vi "Drive Controller.vi"(8 "error in":errorcluster) -> ()   [LabVIEW 2020]
doc: "This VI executes continuously carrying out the current operation and responding to updates or new operation requests. It will often contain the timing or control code that is difficult to place directly in TeleOp. This VI generally opens all sensors and motors and isolates the rest of the robot code from knowing implementation details of how the operations are carried out."
uses:
  Drive Setpoints.ctl
  Drive Operations.ctl
  Robot Velocities.ctl
  <vilib>/Rock Robotics/WPI/ThirdParty/Phoenix-LabVIEW/Motor Controller/Controls/CTRE_Phoenix_MotorControl_ControlMode.ctl
panel:
  in  "milliseconds to wait":u32
  out "Current\nCmd":string
  # "Tip: The graph shows the motor setpoints. It may also be helpful to observe inputs and sensor values.\nYou may also want to display tuning or debugging controls."
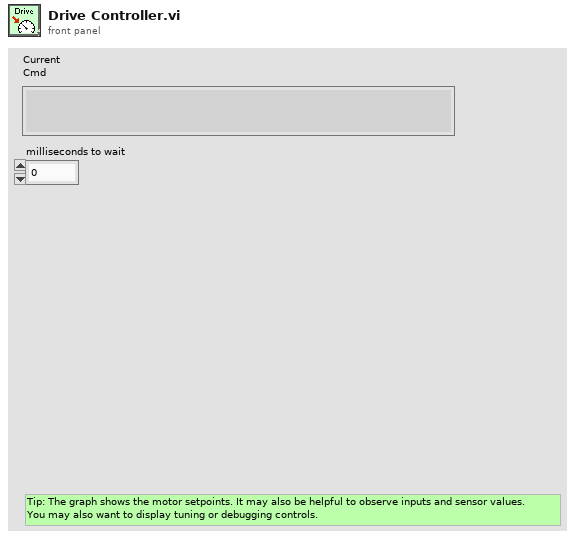
[diagram p1: front panel]
types:
  T1 = cluster{"LF radius":dbl[], "LB radius":dbl[], "RF radius":dbl[], "RB radius":dbl[]}
  T2 = cluster{"LF ID":u8, "LB ID":u8, "RF ID":u8, "RB ID":u8}
  T3 = typedef "Drive Setpoints.ctl" = cluster{"Operation":T4, "Robot Velocities":T5, "Reset Pods?":bool}
  T4 = typedef "Drive Operations.ctl" = enum16{"Reserve", "Read Current", "Immediate", "Calibrate"}
  T5 = typedef "Robot Velocities.ctl" = cluster{"vx":dbl, "vy":dbl, "w":dbl}
  T6 = typedef "Swerve Motors.ctl" = cluster{"Drive Motors":cluster{"Left Front":T7, "Left Back":T7, "Right Front":T7, "Right Back":T7}, "Steer Motors":cluster{"Left Front":T7, "Left Back":T7, "Right Front":T7, "Right Back":T7}}
  T7 = typedef "WPI_MotorControlDeviceRef.ctl" = cluster{"DeviceStatus":errorcluster, "Type":T8, "PWM":cluster{"PWM Channel":T9, "DeadBand":T10}, "CAN":cluster{"Device Number":u8, "SetOutput VI Ref":variant, "GetOutput VI Ref":variant, "Enable VI Ref":variant, "Disable VI Ref":variant, "Data":variant}, "Invert":bool, "DIO PWM":cluster{"PWM \"Enable\" Channel":T9, "DIOChannel":T11, "PWM Rate":dbl}}
  T8 = typedef "WPI_MotorControlType.ctl" = enum16{"PWM", "CAN", "DIO PWM"}
  T9 = typedef "FPGA_DIOPWMChannel.ctl" = enum8{"PWM 0", "PWM 1", "PWM 2", "PWM 3", "PWM 4", "PWM 5", "PWM 6", "PWM 7", "PWM 8", "PWM 9", "PWM MXP 0", "PWM MXP 1", "PWM MXP 2", "PWM MXP 3", "PWM MXP 4", "PWM MXP 5", "PWM MXP 6", "PWM MXP 7", "PWM MXP 8", "PWM MXP 9", "Invalid"}
  T10 = typedef "WPI_PWMDeadband.ctl" = cluster{"Name":string, "maxPositivePwm":i32, "minPositivePwm":i32, "centerPwm":i32, "maxNegativePwm":i32, "minNegativePwm":i32, "angularRange":u16}
  T11 = typedef "FPGA_DIOChannel.ctl" = enum8{"DIO 0", "DIO 1", "DIO 2", "DIO 3", "DIO 4", "DIO 5", "DIO 6", "DIO 7", "DIO 8", "DIO 9", "DIO MXP 0", "DIO MXP 1", "DIO MXP 2", "DIO MXP 3", "DIO MXP 4", "DIO MXP 5", "DIO MXP 6", "DIO MXP 7", "DIO MXP 8", "DIO MXP 9", "DIO MXP 10", "DIO MXP 11", "DIO MXP 12", "DIO MXP 13", "DIO MXP 14", "DIO MXP 15", "SPI Port CS1", "SPI Port CS2", "SPI Port CS3", "SPI Port MISO", "SPI Port MOSI", "Invalid"}
  T12 = typedef "Swerve CANCoders.ctl" = cluster{"Left Front":T13, "Left Back":T13, "Right Front":T13, "Right Back":T13}
  T13 = typedef "CTRE_Phoenix_CANcoder_DeviceRef.ctl" = cluster{"DeviceStatus":errorcluster, "Device Number":u8, "Handle":u64, "UsageFrame":u32, "Library Path":path}
  T14 = typedef "Command Status Info.ctl" = cluster{"Name":string, "Status":T15, "notifier out":T16}
  T15 = typedef "Completion Status.ctl" = enum16{"Successful", "Aborted", "Incomplete"}
  T16 = typedef "Completion Notifier.ctl" = refnum<notifier>
  T17 = cluster{"SubSystem Data":T3, cluster{"Start Time (ms)":u32, "Iterations":i32}, cluster{"Command Info":T14, "Description":string, "Default Command":T3, "queue out":refnum<queue>, "Subsystem Name":string}}
  T18 = cluster{"Left Front":dbl, "Left Back":dbl, "Right Front":dbl, "Right Back":dbl}
  T19 = cluster{"Left Front":i32, "Left Back":i32, "Right Front":i32, "Right Back":i32}
  T20 = typedef "Pod Setpoints.ctl" = cluster{"Left Front":cluster{"Velocity":dbl, "Theta":dbl}, "Left Back":cluster{"Velocity":dbl, "Theta":dbl}, "Right Front":cluster{"Velocity":dbl, "Theta":dbl}, "Right Back":cluster{"Velocity":dbl, "Theta":dbl}}
  T21 = typedef "CTRE_Phoenix_MotorControl_ControlMode.ctl" = u16
  T22 = cluster{"Left Front":T7, "Left Back":T7, "Right Front":T7, "Right Back":T7}
  T23 = cluster{"SubSystem Data":T3, cluster{"Start Time (ms)":u32, "Iterations":i32}, "Default Command Arguments":cluster{"Command Info":T14, "Description":string, "Default Command":T3, "queue out":refnum<queue>, "Subsystem Name":string}}
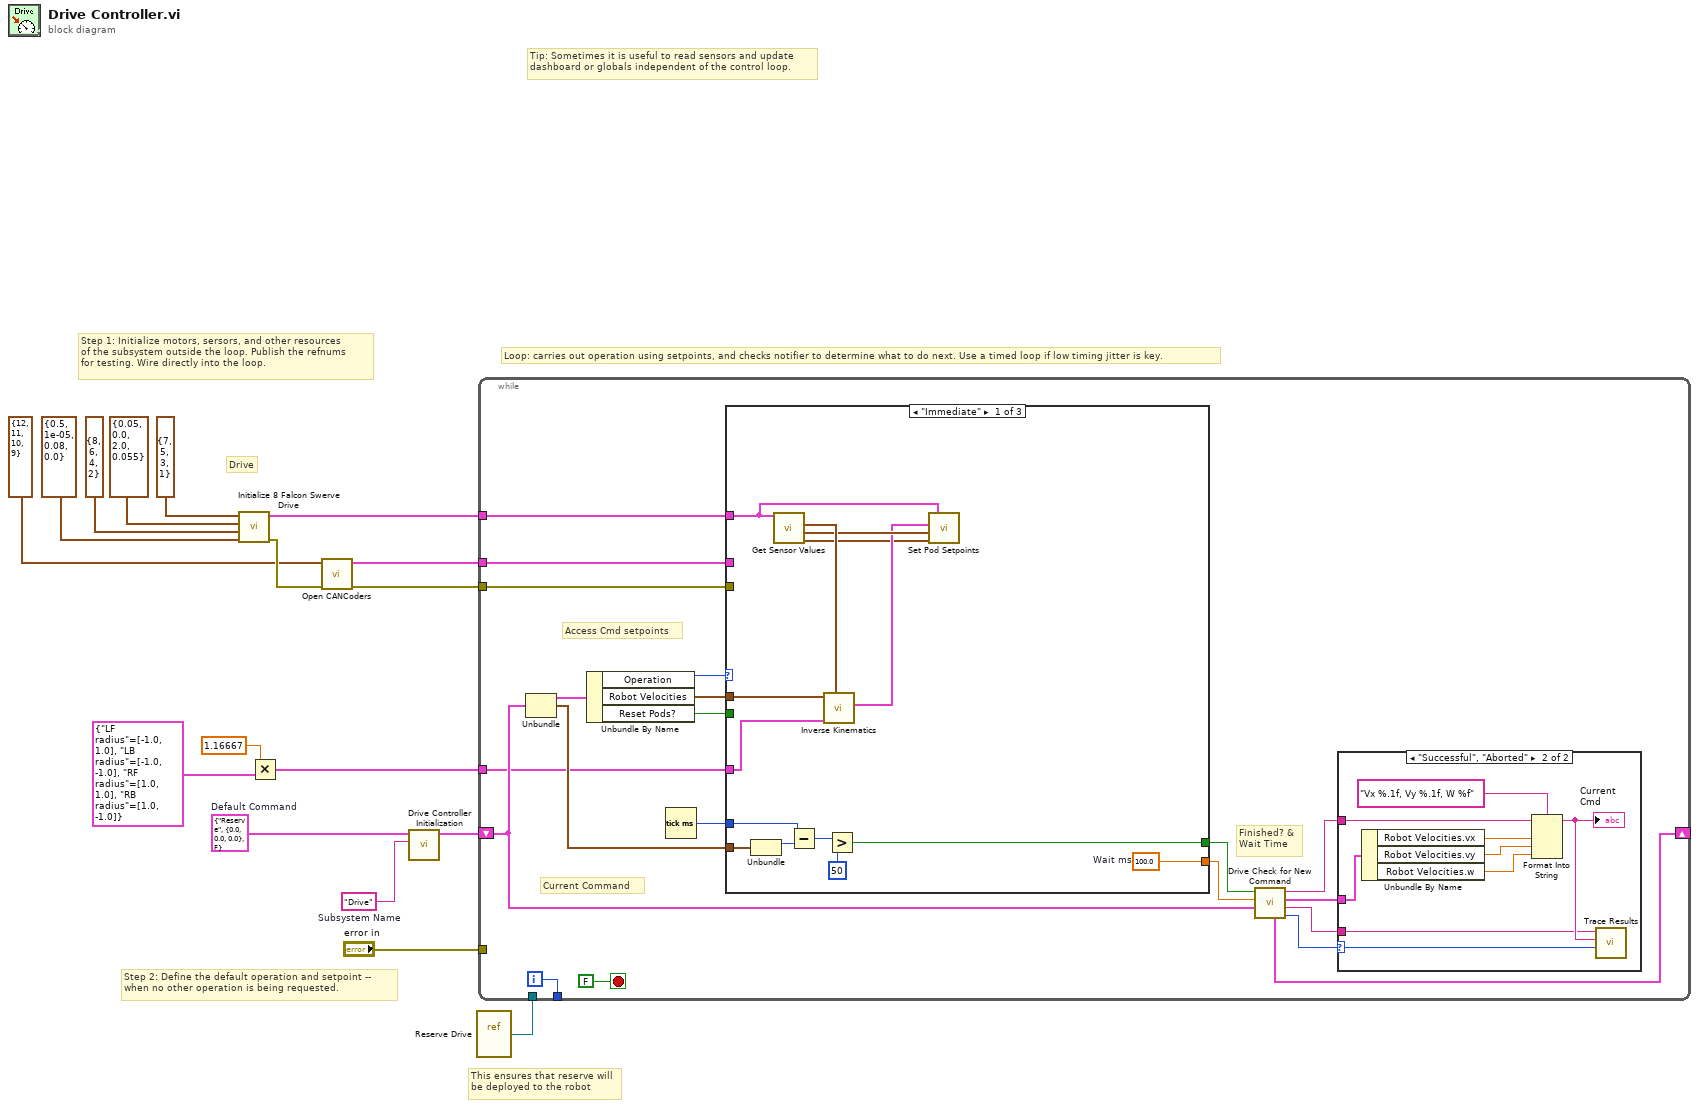
[diagram p0: block diagram]
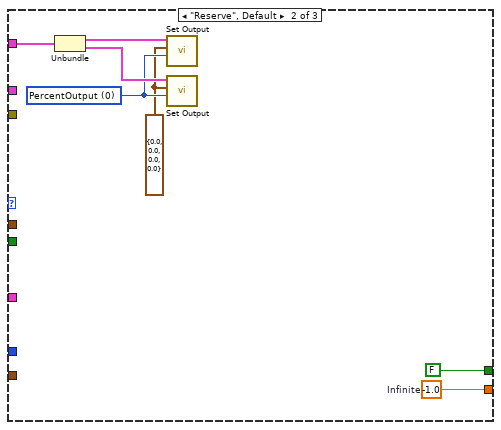
[diagram p3: hidden frame]
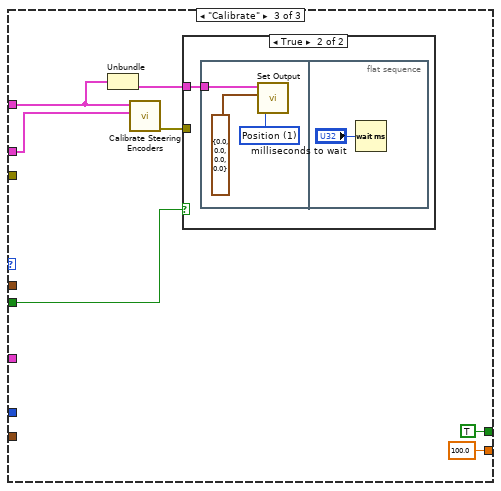
[diagram p4: hidden frame]
diagram:
  w13 = T3 {"Operation"=enum."Reserve", "Robot Velocities"={"vx"=0.0, "vy"=0.0, "w"=0.0}, "Reset Pods?"=FALSE}  # Default Command
  w17 = "Drive"  # Subsystem Name
  # "Drive"
  # "This ensures that reserve will\nbe deployed to the robot"
  # "Tip: Sometimes it is useful to read sensors and update\ndashboard or globals independent of the control loop."
  # "Step 2: Define the default operation and setpoint --\nwhen no other operation is being requested."
  # "Step 1: Initialize motors, sersors, and other resources\nof the subsystem outside the loop. Publish the refnums\nfor testing. Wire directly into the loop."
  # "Loop: carries out operation using setpoints, and checks notifier to determine what to do next. Use a timed loop if low timing jitter is key."
  n1 = call "Initialize 8 Falcon Swerve Drive.vi"("Steer PIDF"=cluster{"P":dbl, "I":dbl, "D":dbl, "F":dbl} {"P"=0.5, "I"=1e-05, "D"=0.08, "F"=0.0} ("PIDF"), "Steer CAN IDs"=T2 {"LF ID"=8, "LB ID"=6, "RF ID"=4, "RB ID"=2} ("Can IDs"), "Drive PIDF"=cluster{"P":dbl, "I":dbl, "D":dbl, "F":dbl} {"P"=0.05, "I"=0.0, "D"=2.0, "F"=0.055} ("PIDF"), "Drive CAN IDs"=T2 {"LF ID"=7, "LB ID"=5, "RF ID"=3, "RB ID"=1} ("Can IDs")) -> ("error out"=w7:errorcluster, "Motors"=w8:T6)  [unwired: 6 in]
  n2 = Multiply(x=1.16667, y=T1 {"LF radius"=[-1.0, 1.0], "LB radius"=[-1.0, -1.0], "RF radius"=[1.0, 1.0], "RB radius"=[1.0, -1.0]} ("Radii")) -> (x*y=w1:T1)
  n3 = call "Open CANCoders.vi"("error in"=w7, "CANCoder Can IDs"=T2 {"LF ID"=12, "LB ID"=11, "RF ID"=10, "RB ID"=9}) -> ("error out"=w4:errorcluster, "CANCoders"=w5:T12)  [unwired: 8 in]
  n4 = call "Drive Controller Initialization.vi"("Subsystem Name"=w17, "Default Command"=w13) -> ("Current Command"=w15:T17)  [unwired: 9 in]
  n5 = vi-ref "Reserve Drive.vi"() -> (w14:refnum<vi>)
  n6 = while {
    shift-right: [w31] -> _
    shift-left: w15 -> [w24]
    tunnel: [w36] -> _
    tunnel: "error in" -> [_]
    tunnel: w14 -> [_]
    tunnel: w8 -> [w22]
    tunnel: w5 -> [w21]
    tunnel: w4 -> [w20]
    tunnel: w1 -> [w18]
    i -> [w36]
    stop <- FALSE stop-if-true
    # "Current Command"
    # "Access Cmd setpoints"
    # "Finished? &\nWait Time"
    n7 = Unbundle(w24) -> ("SubSystem Data"=w35:T3, w25:cluster{"Start Time (ms)":u32, "Iterations":i32})  [unwired: 1 out]
    n8 = Unbundle By Name(w35) -> ("Operation"=w34:T4, "Robot Velocities"=w23:T5, "Reset Pods?"=w19:bool)
    n9 = Tick Count (ms)() -> (millisecond timer value=w33:u32)
    n10 = case shown="\"Immediate\"" w34 {
      tunnel: [w60 w67 100.0 ("Infinite")] -> w30
      tunnel: [w47 FALSE ("ignore previous (F)") TRUE ("ignore previous (F)")] -> w29
      tunnel: w25 -> [w52 _ _]
      tunnel: w33 -> [w51 _ _]
      tunnel: w23 -> [w59 _ _]
      tunnel: w22 -> [w54 w65 w72]
      tunnel: w21 -> [_ _ w74]
      tunnel: w20 -> [_ _ _]
      tunnel: w19 -> [_ _ w70]
      tunnel: w18 -> [w58 _ _]
      frame "Immediate" {
        w60 = 100.0  # Wait ms
        n11 = Unbundle(w52) -> ("Start Time (ms)"=w50:u32)  [unwired: 1 out]
        n12 = call "Get Sensor Values.vi"("Motors"=w54) -> ("Steer Angles (ticks)"=w53:T19, "Drive Velocities (ticks/ds)"=w56:T19, "Steer Angles (degrees)"=w57:T19)  [unwired: 7 in, 1 out]
        n13 = Subtract(x=w51, y=w50) -> (x-y=w49:u32)
        n14 = call "Inverse Kinematics.vi"("Current Pod Steering (deg)"=w57, "Radii (ft)"=w58, "Target Velocity (ft/s and deg/s)"=w59) -> ("Pod Setpoints (ft/s and deg)"=w55:T20)  [unwired: 5 in, 3 out]
        n15 = Greater?(x=w49, y=u32 50) -> (0:w47:bool)
        n16 = call "Set Pod Setpoints.vi"("Steer Angles (ticks)"=w53, "Drive Velocities (ticks/ds)"=w56, "Pod Setpoints (ft/s and deg)"=w55, "Motors"=w54) -> ()  [unwired: 8 in]
      }
      frame "Reserve", Default {
        w61 = T18 {"Left Front"=0.0, "Left Back"=0.0, "Right Front"=0.0, "Right Back"=0.0} ("Setpoints")
        w62 = T21 0 items=["PercentOutput"=0, "Position"=1, "Velocity"=2, "Current"=3, "Follower"=5, "MotionProfile"=6, "MotionMagic"=7, "MotionProfileArc"=10, "Disabled"=15] ("Control Mode")
        w67 = -1.0  # Infinite
        n17 = Unbundle(w65) -> ("Drive Motors"=w63:T22, "Steer Motors"=w64:T22)
        n18 = call "Set Output.vi"("Control Mode"=w62, "Setpoints"=w61, "Motors"=w63) -> ()  [unwired: 9 in]
        n19 = call "Set Output.vi"("Control Mode"=w62, "Setpoints"=w61, "Motors"=w64) -> ()  [unwired: 9 in]
      }
      frame "Calibrate" {
        n20 = Unbundle(w72) -> ("Steer Motors"=w71:T22)  [unwired: 1 out]
        n21 = call "Calibrate Steering Encoders.vi"("CANCoders"=w74, "Motors"=w72) -> ("error out"=w68:errorcluster)  [unwired: 8 in, 1 out]
        n22 = case shown="True" w70 {
          tunnel: w71 -> [_ w75]
          tunnel: w68 -> [_ _]
          frame False {
          }
          frame True {
            n23 = flat-sequence {
              tunnel: w75 -> [w77]
              frame #0 {
                w76 = T21 1 items=["PercentOutput"=0, "Position"=1, "Velocity"=2, "Current"=3, "Follower"=5, "MotionProfile"=6, "MotionMagic"=7, "MotionProfileArc"=10, "Disabled"=15] ("Control Mode")
                n24 = call "Set Output.vi"("Control Mode"=w76, "Setpoints"=T18 {"Left Front"=0.0, "Left Back"=0.0, "Right Front"=0.0, "Right Back"=0.0}, "Motors"=w77) -> ()  [unwired: 9 in]
              }
              frame #1 {
                n25 = Wait (ms)(milliseconds to wait="milliseconds to wait") -> ()  [unwired: 1 out]
              }
            }
          }
        }
      }
    }
    n26 = call "Drive Check for New Command.vi"("input cluster"=w24, "Wait time (ms)"=w30, "Finished?"=w29) -> ("Completion"=w32:T15, "Subsystem Name"=w26:string, "Current Command"=w27:T3, "Initial Trace String"=w28:string, "Next Command"=w31:T23)  [unwired: 4 in]
    n27 = case shown="\"Successful\", \"Aborted\"" w32 {
      selector: w32 -> [_ w46]
      tunnel: w28 -> [_ w41]
      tunnel: w27 -> [_ w42]
      tunnel: w26 -> [_ w38]
      frame "Incomplete", Default {
        # "Continuing current command"
      }
      frame "Successful", "Aborted" {
        # "Report and setup for next command"
        n28 = Unbundle By Name(w42) -> ("Robot Velocities.vx"=w44:dbl, "Robot Velocities.vy"=w45:dbl, "Robot Velocities.w"=w39:dbl)
        n29 = Format Into String(format string="Vx %.1f, Vy %.1f, W %f", initial string=w41, w44, w45, w39) -> (resulting string=w40:string)  [unwired: 1 in, 1 out]
        "Current\nCmd" <- w40
        n30 = call <vilib>:"Trace Results.vi"("Status of previous command"=w46, "Description"=w40, "Subsystem"=w38) -> ()  [unwired: 9 in]
      }
    }
  }
